vi "sub_sample_without_replacement.vi"(8 "error in (no error)":errorcluster, 9 "number of unique samples":i32, 10 "probability":dbl[](array[numeric]), 11 "List":i32[](array[numeric])=[0, 0, 0, 0, 0, 0, 0, 0, 0, 0]) -> (0 "error out":errorcluster, 2 "probability not equal to 1":bool, 3 "unique samples":i32[](array[numeric]))   [LabVIEW 2010]
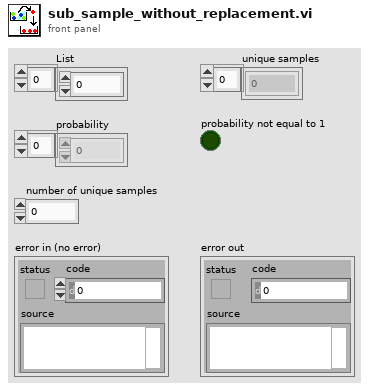
[diagram p1: front panel]
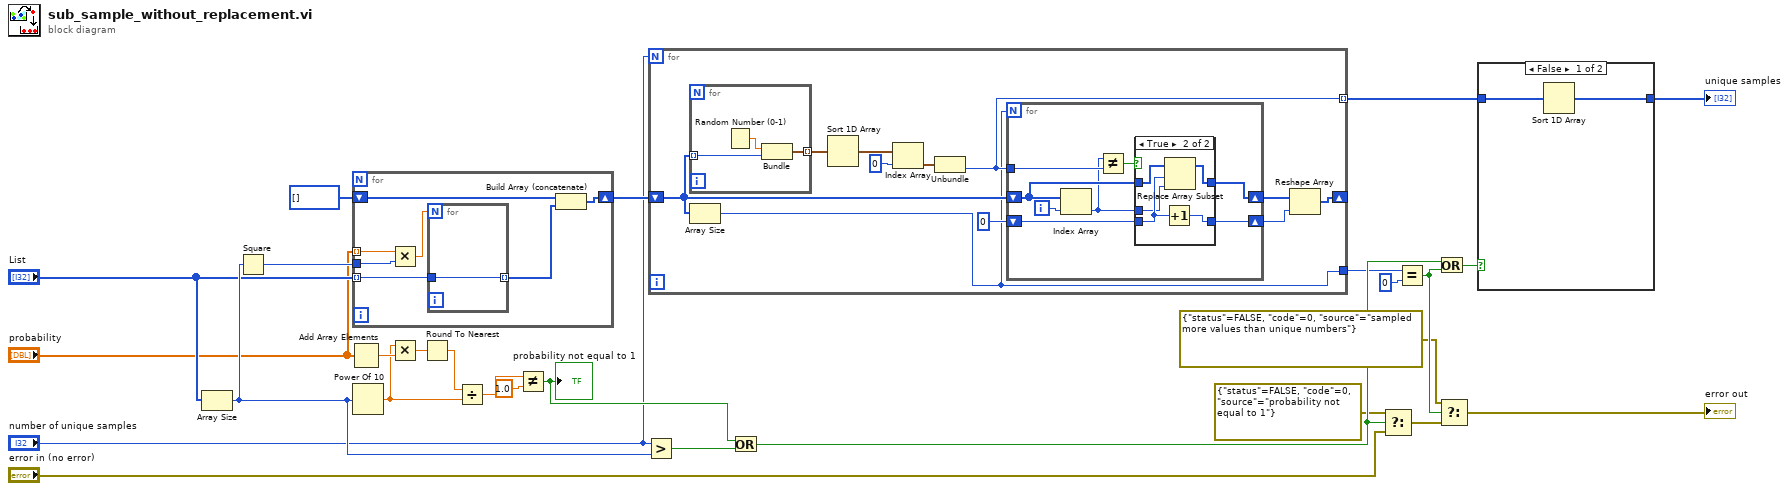
[diagram p0: block diagram]
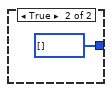
[diagram p2: hidden frame]
diagram:
  n1 = Array Size(array="List") -> (size(s)=w13:i32)
  n2 = Square(x=w13) -> (x^2=w8:i32)
  n3 = Add Array Elements(numeric array="probability") -> (sum=w7:dbl)
  n4 = for {
    tunnel: "probability" -> [w34] mode=indexing
    tunnel: "List" -> [w32] mode=indexing
    shift-right: [w30] -> w17
    shift-left: i32[] [] -> [w29]
    tunnel: w8 -> [w28]
    n5 = Multiply(x=w34, y=w28) -> (x*y=w33:dbl)
    n6 = for {
      N: w33 -> [_]
      tunnel: w32 -> [w35]
      tunnel: [w35] -> w31 mode=indexing
    }
    n7 = Build Array (concatenate)(w29, w31) -> (w30:i32[])
  }
  n8 = Power Of 10(x=w13) -> (10^x=w6:dbl)
  n9 = Multiply(x=w6, y=w7) -> (x*y=w4:dbl)
  n10 = Round To Nearest(number=w4) -> (nearest integer value=w5:dbl)
  n11 = Divide(x=w5, y=w6) -> (x/y=w9:dbl)
  n12 = Not Equal?(x=w9, y=1.0) -> (x != y?=w15:bool)
  "probability not equal to 1" <- w15
  n13 = Greater?(x="number of unique samples", y=w13) -> (0:w14:bool)
  n14 = for {
    N: "number of unique samples" -> [_]
    tunnel: [w39] -> w24 mode=indexing
    shift-right: [w38] -> _
    shift-left: w17 -> [w37]
    tunnel: [w36] -> w20
    n15 = for {
      tunnel: [w64] -> w46 mode=indexing
      tunnel: w37 -> [w62] mode=indexing
      n16 = Random Number (0-1)() -> (number: 0 to 1=w63:dbl)
      n17 = Bundle("number: 0 to 1"=w63, w62) -> (w64:cluster{"number: 0 to 1":dbl, i32})  [unwired: 1 out]
    }
    n18 = Array Size(array=w37) -> (size(s)=w36:i32)
    n19 = Sort 1D Array(array=w46) -> (sorted array=w45:cluster{"number: 0 to 1":dbl, i32}[])
    n20 = Index Array(array=w45, index=0) -> (element=w44:cluster{"number: 0 to 1":dbl, i32})
    n21 = Unbundle(w44) -> (w39:i32)  [unwired: 1 out]
    n22 = for {
      N: w36 -> [_]
      shift-right: [w54] -> w41
      shift-left: w37 -> [w52]
      shift-right: [w50] -> w40
      shift-left: 0 -> [w51]
      tunnel: w39 -> [w49]
      i -> [w53]
      n23 = Index Array(array=w52, index=w53) -> (element=w47:i32)
      n24 = Not Equal?(x=w47, y=w49) -> (x != y?=w48:bool)
      n25 = case shown="True" w48 {
        tunnel: w52 -> [w56 w61]
        tunnel: [w56 w60] -> w54
        tunnel: w51 -> [w55 w59]
        tunnel: [w55 w58] -> w50
        tunnel: w47 -> [_ w57]
        frame False {
        }
        frame True {
          n26 = Increment(x=w59) -> (x+1=w58:i32)
          n27 = Replace Array Subset(array=w61, new element=w57, index=w59) -> (w60:i32[])
        }
      }
    }
    n28 = Reshape Array(w41, w40) -> (w38:i32[])
  }
  n29 = Or(x=w15, y=w14) -> (x .or. y?=w25:bool)
  n30 = Select(t=errorcluster {"status"=FALSE, "code"=0, "source"="probability not equal to 1"} ("error constant"), s=w25, f="error in (no error)") -> (s? t:f=w22:errorcluster)
  n31 = Equal?(x=w20, y=0) -> (x = y?=w26:bool)
  n32 = Or(x=w25, y=w26) -> (x .or. y?=w27:bool)
  n33 = Select(t=errorcluster {"status"=FALSE, "code"=0, "source"="sampled more values than unique numbers"} ("error constant"), s=w26, f=w22) -> (s? t:f=→"error out":errorcluster)
  n34 = case shown="False" w27 {
    tunnel: [w65 i32[] []] -> w23
    tunnel: w24 -> [w66 _]
    frame False {
      n35 = Sort 1D Array(array=w66) -> (sorted array=w65:i32[])
    }
    frame True {
    }
  }
  "unique samples" <- w23
